vi "Find All Zeroes Inner Part.vi"(3 "accuracy":dbl=1e-08 format="%.2e", 4 "algorithm":u16, 5 "formula":string, 6 "X and Y values":cluster{"X Values":dbl[], "Y Values":dbl[]} {"Y Values" format="%.2f"; "X Values" format="%.2f"}) -> (0 "error":i32, 1 "f(Zeroes)":dbl[](array[numeric]) format="%.2f", 2 "Zeroes":dbl[](array[numeric]) format="%.2f")   [LabVIEW 2010, in "NI_Gmath.lvlib"]
uses:
  NI_Gmath.lvlib
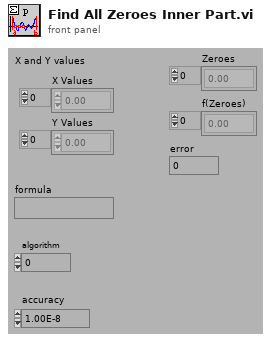
[diagram p1: front panel]
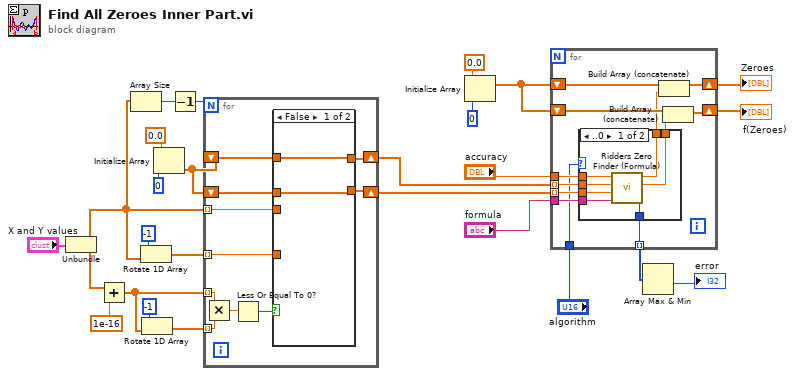
[diagram p0: block diagram]
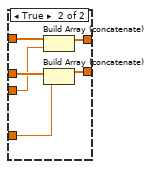
[diagram p2: hidden frame]
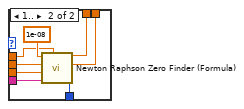
[diagram p3: hidden frame]
diagram:
  n1 = Unbundle("X and Y values") -> ("X Values"=w12:dbl[], "Y Values"=w6:dbl[])
  n2 = Add(x=w6, y=1e-16) -> (x+y=w8:dbl[])
  n3 = Array Size(array=w12) -> (size(s)=w2:i32)
  n4 = Rotate 1D Array(1:w12, 2:-1) -> (0:w14:dbl[])
  n5 = Rotate 1D Array(1:w8, 2:-1) -> (0:w5:dbl[])
  n6 = Initialize Array(0.0, 0) -> (w11:dbl[])
  n7 = Decrement(x=w2) -> (x-1=w3:i32)
  n8 = for {
    N: w3 -> [_]
    tunnel: w8 -> [w36] mode=indexing
    tunnel: w5 -> [w35] mode=indexing
    shift-right: [w31] -> w1
    shift-left: w11 -> [w32]
    shift-right: [w29] -> w20
    shift-left: w11 -> [w30]
    tunnel: w12 -> [w28] mode=indexing
    tunnel: w14 -> [w27] mode=indexing
    n9 = Multiply(x=w36, y=w35) -> (x*y=w34:dbl)
    n10 = Less Or Equal To 0?(x=w34) -> (x <= 0?=w33:bool)
    n11 = case shown="False" w33 {
      tunnel: w32 -> [w38 w44]
      tunnel: [w38 w43] -> w31
      tunnel: w30 -> [w37 w42]
      tunnel: [w37 w41] -> w29
      tunnel: w28 -> [_ w40]
      tunnel: w27 -> [_ w39]
      frame False {
      }
      frame True {
        n12 = Build Array (concatenate)(w44, w40) -> (w43:dbl[])
        n13 = Build Array (concatenate)(w42, w39) -> (w41:dbl[])
      }
    }
  }
  n14 = Initialize Array(0.0, 0) -> (w19:dbl[])
  n15 = for {
    tunnel: w1 -> [w50] mode=indexing
    tunnel: w20 -> [w49] mode=indexing
    tunnel: "accuracy" -> [w47]
    tunnel: "formula" -> [w48]
    shift-right: [w53] -> w24
    shift-left: w19 -> [w56]
    shift-right: [w54] -> w25
    shift-left: w19 -> [w55]
    tunnel: "algorithm" -> [w46]
    tunnel: [w45] -> w23 mode=indexing
    n16 = case shown="..0" w46 {
      tunnel: w47 -> [w63 w70]
      tunnel: w48 -> [w60 w67]
      tunnel: w49 -> [w61 w68]
      tunnel: w50 -> [w62 w69]
      tunnel: [w58 w65] -> w51
      tunnel: [w59 w66] -> w52
      tunnel: [w57 w64] -> w45
      frame ..0 {
        n17 = call "Ridders Zero Finder (Formula).vi"("formula"=w60, "end"=w61, "start"=w62, "accuracy"=w63) -> ("error"=w57:i32, "f(zero)"=w58:dbl, "zero"=w59:dbl)  [unwired: 5 out]
      }
      frame 1.. {
        n18 = call "Newton Raphson Zero Finder (Formula).vi"("accuracy"=w70, "formula"=w67, "end"=w68, "start"=w69, "h"=1e-08) -> ("error"=w64:i32, "f(zero)"=w65:dbl, "zero"=w66:dbl)  [unwired: 4 out]
      }
    }
    n19 = Build Array (concatenate)(w56, w52) -> (w53:dbl[])
    n20 = Build Array (concatenate)(w55, w51) -> (w54:dbl[])
  }
  "f(Zeroes)" <- w25
  "Zeroes" <- w24
  n21 = Array Max & Min(array=w23) -> (min value=→"error":i32)  [unwired: 3 out]
